vi "Enable or Disable UI Elements.vi"(8 "error in (no error)":errorcluster, 10 "Enable?":bool, 11 "UI Refs in":T1) -> (0 "error out":errorcluster, 3 "UI Refs out":T1)   [LabVIEW 2016, in "System Mapping Tool.lvlib"]
uses:
  System Mapping Tool.lvlib
  TypeDefs/UI Refs.ctl
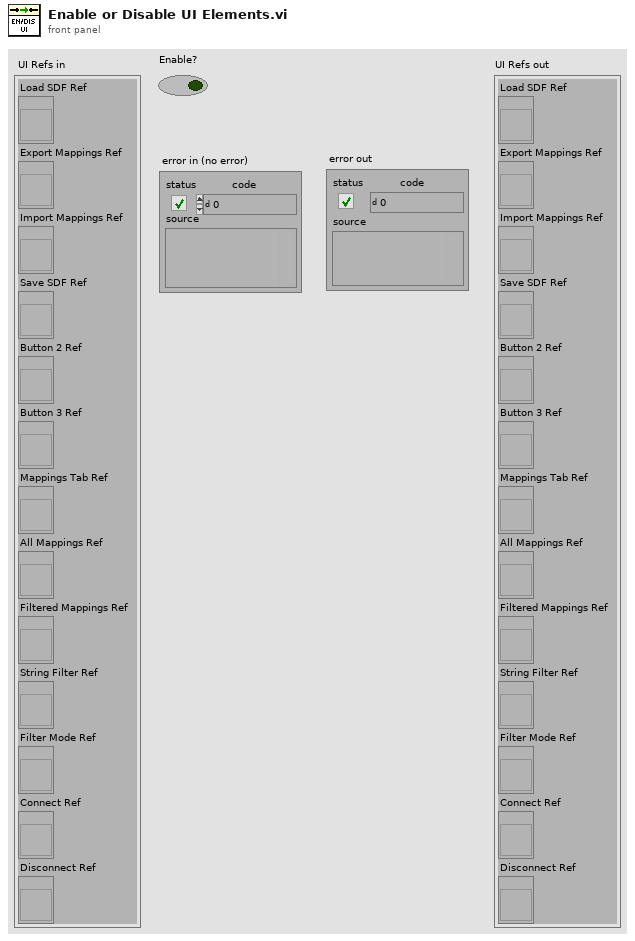
[diagram p1: front panel]
types:
  T1 = typedef "System Mapping Tool.lvlib/UI Refs.ctl" = cluster{"Load SDF Ref":refnum<vi>, "Export Mappings Ref":refnum<vi>, "Import Mappings Ref":refnum<vi>, "Save SDF Ref":refnum<vi>, "Button 2 Ref":refnum<vi>, "Button 3 Ref":refnum<vi>, "Mappings Tab Ref":refnum<vi>, "All Mappings Ref":refnum<vi>, "Filtered Mappings Ref":refnum<vi>, "String Filter Ref":refnum<vi>, "Filter Mode Ref":refnum<vi>, "Connect Ref":refnum<vi>, "Disconnect Ref":refnum<vi>}
  T2 = enum8{"Enabled", "Disabled", "Disabled and Grayed Out"}
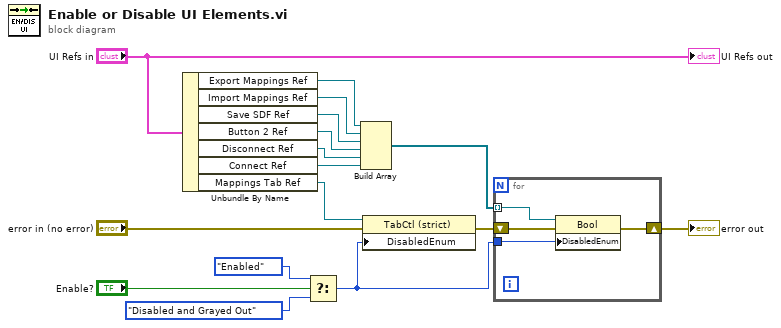
[diagram p0: block diagram]
diagram:
  n1 = Unbundle By Name("UI Refs in") -> ("Export Mappings Ref"=w13:refnum<vi>, "Import Mappings Ref"=w14:refnum<vi>, "Save SDF Ref"=w15:refnum<vi>, "Button 2 Ref"=w16:refnum<vi>, "Disconnect Ref"=w1:refnum<vi>, "Connect Ref"=w2:refnum<vi>, "Mappings Tab Ref"=w11:refnum<vi>)
  n2 = Select(t=T2."Enabled" ("Disabled"), s="Enable?", f=T2."Disabled and Grayed Out" ("Disabled")) -> (s? t:f=w5:T2)
  n3 = Build Array(w13, w14, w15, w16, w1, w2) -> (w6:refnum<vi>[])
  n4 = property class="TabCtl (strict)"(reference=w11, error in="error in (no error)", "DisabledEnum"=w5) -> (error out=w7:errorcluster)  [unwired: 1 out]
  n5 = for {
    shift-right: [w19] -> w4
    shift-left: w7 -> [w20]
    tunnel: w6 -> [w18] mode=indexing
    tunnel: w5 -> [w17]
    n6 = property class="Bool"(reference=w18, error in=w20, "DisabledEnum"=w17) -> (error out=w19:errorcluster)  [unwired: 1 out]
  }
  "error out" <- w4
  "UI Refs out" <- "UI Refs in"
